vi "ReadJoystick.vi"(0 "Joystick Number (1)":u8(ring)=1 items=["1"=1, "2"=2], 1 "Remote (1)":u8(ring)=1 items=["1"=1, "2"=2]) -> (2 "POV":T1 items=["None"=-1, "POV Up"=0, "POV Up Right"=1, "POV Right"=2, "POV Down Right"=3, "POV Down"=4, "POV Down Left"=5, "POV Left"=6, "POV Up Left"=7], 3 "Y Axis":i8, 4 "X Axis":i8)   [LabVIEW 2010, in "FTC.lvlib" / "Remote Interface.lvlib"]
uses:
  Remote Interface.lvlib
  <vilib>/FTC/FTC POVState.ctl
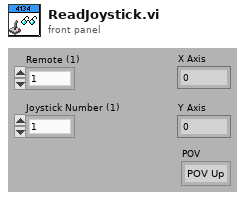
[diagram p1: front panel]
types:
  T1 = typedef "FTC POVState.ctl" = i8
  T2 = typedef "FTC ControllerState.ctl" = cluster{"Left X":i8, "Left Y":i8, "Right X":i8, "Right Y":i8, "Button Encoding 9-12":u8, "Button Encoding 1-8":u8, "POV":T1}
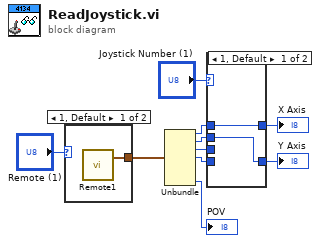
[diagram p0: block diagram]
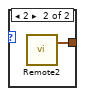
[diagram p3: hidden frame]
diagram:
  n1 = case shown="1, Default" "Remote (1)" {
    tunnel: [w11 w12] -> w6
    frame 1, Default {
      n2 = call "Remote1.vi"() -> ("Controller State"=w11:T2)  [unwired: 4 in]
    }
    frame 2 {
      n3 = call "Remote2.vi"() -> ("Controller State"=w12:T2)  [unwired: 4 in]
    }
  }
  n4 = Unbundle(w6) -> ("Left X"=w5:i8, "Left Y"=w4:i8, "Right X"=w3:i8, "Right Y"=w2:i8, "POV"=→"POV":T1)  [unwired: 2 out]
  n5 = case shown="1, Default" "Joystick Number (1)" {
    tunnel: w2 -> [_ w15]
    tunnel: w3 -> [_ w16]
    tunnel: w4 -> [w13 _]
    tunnel: w5 -> [w14 _]
    tunnel: [w14 w16] -> w8
    tunnel: [w13 w15] -> w7
    frame 1, Default {
    }
    frame 2 {
    }
  }
  "X Axis" <- w8
  "Y Axis" <- w7
